vi "Stepper.vi"(0 "VISA resource name":refnum<visa-resource-name>="COM1", 1 "baud rate":u32=9600, 2 "data bits":u16=8 min=5 max=8 step=1, 3 "parity":u16(ring) items=["None", "Odd", "Even", "Mark", "Space"], 4 "stop bits":u16(ring)=10 items=["1.0"=10, "1.5"=15, "2.0"=20], 7 "flow control":u16(ring) items=["None"=0, "XON/XOFF"=1, "RTS/CTS"=2, "DTR/DSR"=4]) -> ()   [LabVIEW 2015]
doc: "The Basic Serial Read and Write example performs a Serial Port Read, a Serial Port Write, or a combination of these actions. The user selects the actions (read or write) on the front panel. If both are selected, the VI will write the data first, read data, and then close the VISA session that is opened to the port. This VI will wait until the specified number of bytes is received at the port. Only the number of bytes specified will be read.\n\nINSTRUCTIONS:\n1) Select the serial resource and configuration parameters (baud rate, data bits, parity, stop bits, flow control).\n2) Select the operations to be performed. \n3) Connect the serial port to your device. If no device is available, perform a loopback test by doing one of the following. Short pins 2 and 3 on a RS-232 cable or short pin 4 to pin 8 and pin 5 to pin 9 on a RS-485/422 cable. \n4) Run the VI to see the data read. (The \"read string\" will match the \"string to write\" if a loopback test was performed.)\n\nNote: The parameters set for the serial port must match the parameters of the connected instrument or device. In this example, the bytes to read parameter specifies the number of bytes that the serial port reads. If there were more bytes at the port than the number specified in bytes to read, those bytes would not be read. Also, if you specify to read more bytes than the number of bytes actually read, you might receive a timeout error message.\n\nOn the block diagram, the Configure Serial Port VI sets the configuration parameters. The front panel displays the controls used to configure the basic parameters, such as baud rate, data bits, and parity. Constants configure the other parameters the user probably does not need set. After the VISA Configure Serial Port VI opens the VISA session and configures the port, the VI passes the VISA resource name to other VIs that perform operations on that VISA resource. The VISA Write function sends a command to the serial device and the VISA Read function returns data based on the command. The VISA Close function then closes the reference to the serial device. It is important to close the reference; otherwise communication through with that port through protocols other than VISA might not be possible."
uses:
  <vilib>/Instr/_visa.llb/VISA Configure Serial Port (Instr).vi
panel:
  in  "?":string
  in  "Enable":bool
  in  "Clear 6":bool
  in  "Stop All":bool
  in  "Clear 5":bool
  in  "Direction 2":bool
  in  "Clear 4":bool
  in  "Direction 1":bool
  in  "Clear 3":bool
  in  "1/2  Step":bool
  in  "Clear 2":bool
  in  "Clear 1":bool
  in  "1/4 Step":bool
  in  "Reset The System":bool
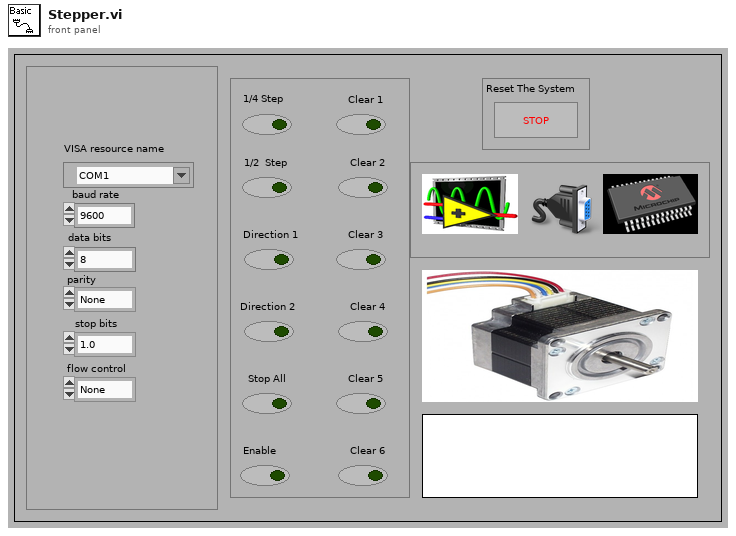
[diagram p1: front panel]
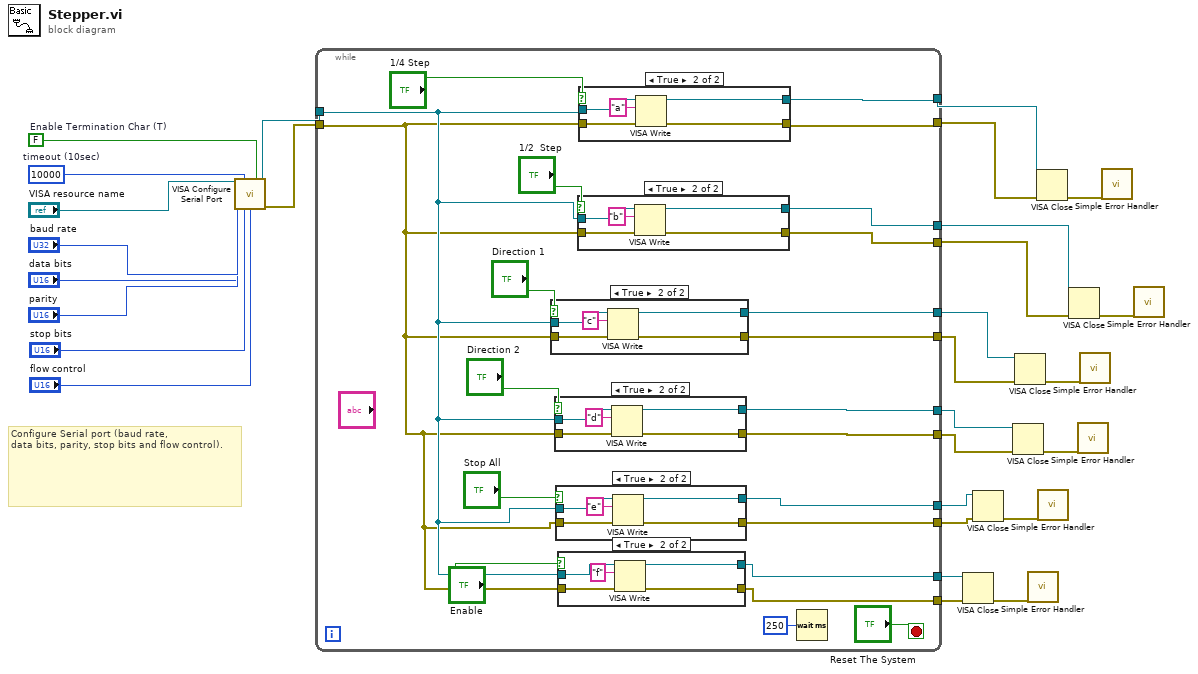
[diagram p0: block diagram]
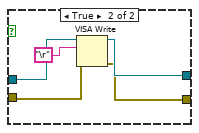
[diagram p3: hidden frame]
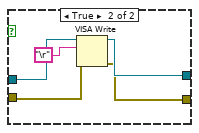
[diagram p5: hidden frame]
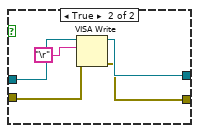
[diagram p7: hidden frame]
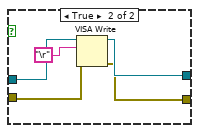
[diagram p9: hidden frame]
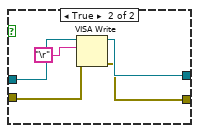
[diagram p11: hidden frame]
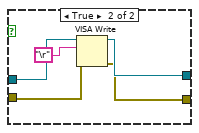
[diagram p13: hidden frame]
diagram:
  w21 = FALSE  # Enable Termination Char (T)
  w22 = u32 10000  # timeout (10sec)
  # "Configure Serial port (baud rate,\ndata bits, parity, stop bits and flow control)."
  n1 = call-poly "VISA Configure Serial Port"("VISA resource name"="VISA resource name", "timeout (10sec)"=w22, "Enable Termination\nChar (T)"=w21, "baud rate (9600)"="baud rate", "data bits (8)"="data bits", "parity (0:none)"="parity", "stop bits (10: 1 bit)"="stop bits", "flow control (0:none)"="flow control") -> ("VISA resource name out"=w25:refnum<visa-resource-name>, "error out"=w26:errorcluster)  [unwired: 6 in]
  n2 = while {
    tunnel: w26 -> [w33]
    tunnel: w25 -> [w34]
    tunnel: [w45] -> w17
    tunnel: [w47] -> w16
    tunnel: [w44] -> w14
    tunnel: [w43] -> w13
    tunnel: [w40] -> w10
    tunnel: [w39] -> w9
    tunnel: [w38] -> w8
    tunnel: [w37] -> w7
    tunnel: [w32] -> w4
    tunnel: [w31] -> w3
    tunnel: [w30] -> w2
    tunnel: [w29] -> w1
    stop <- "Reset The System" stop-if-true
    n3 = case shown="True" "Direction 1" {
      tunnel: [w102 w118] -> w40
      tunnel: w34 -> [w104 w117]
      tunnel: w33 -> [w105 w115]
      tunnel: [w103 w116] -> w39
      frame False {
        n4 = case shown="False" "Clear 3" {
          tunnel: w105 -> [w107 w113]
          tunnel: w104 -> [w108 w112]
          tunnel: [w108 w110] -> w103
          tunnel: [w107 w109] -> w102
          frame False {
          }
          frame True {
            n5 = VISA Write(VISA resource name=w112, write buffer="\r", error in (no error)=w113) -> (VISA resource name out=w110:refnum<visa-resource-name>, error out=w109:errorcluster)  [unwired: 1 out]
          }
        }
      }
      frame True {
        n6 = VISA Write(VISA resource name=w117, write buffer="c", error in (no error)=w115) -> (VISA resource name out=w116:refnum<visa-resource-name>, error out=w118:errorcluster)  [unwired: 1 out]
      }
    }
    n7 = case shown="True" "Direction 2" {
      tunnel: [w85 w101] -> w37
      tunnel: w34 -> [w87 w100]
      tunnel: w33 -> [w88 w98]
      tunnel: [w86 w99] -> w38
      frame False {
        n8 = case shown="False" "Clear 4" {
          tunnel: w88 -> [w90 w96]
          tunnel: w87 -> [w91 w95]
          tunnel: [w91 w93] -> w86
          tunnel: [w90 w92] -> w85
          frame False {
          }
          frame True {
            n9 = VISA Write(VISA resource name=w95, write buffer="\r", error in (no error)=w96) -> (VISA resource name out=w93:refnum<visa-resource-name>, error out=w92:errorcluster)  [unwired: 1 out]
          }
        }
      }
      frame True {
        n10 = VISA Write(VISA resource name=w100, write buffer="d", error in (no error)=w98) -> (VISA resource name out=w99:refnum<visa-resource-name>, error out=w101:errorcluster)  [unwired: 1 out]
      }
    }
    n11 = case shown="True" "Stop All" {
      tunnel: [w51 w67] -> w31
      tunnel: w34 -> [w53 w66]
      tunnel: w33 -> [w54 w64]
      tunnel: [w52 w65] -> w32
      frame False {
        n12 = case shown="False" "Clear 5" {
          tunnel: w54 -> [w56 w62]
          tunnel: w53 -> [w57 w61]
          tunnel: [w57 w59] -> w52
          tunnel: [w56 w58] -> w51
          frame False {
          }
          frame True {
            n13 = VISA Write(VISA resource name=w61, write buffer="\r", error in (no error)=w62) -> (VISA resource name out=w59:refnum<visa-resource-name>, error out=w58:errorcluster)  [unwired: 1 out]
          }
        }
      }
      frame True {
        n14 = VISA Write(VISA resource name=w66, write buffer="e", error in (no error)=w64) -> (VISA resource name out=w65:refnum<visa-resource-name>, error out=w67:errorcluster)  [unwired: 1 out]
      }
    }
    n15 = case shown="True" "Enable" {
      tunnel: [w68 w84] -> w29
      tunnel: w34 -> [w70 w83]
      tunnel: w33 -> [w71 w81]
      tunnel: [w69 w82] -> w30
      frame False {
        n16 = case shown="False" "Clear 6" {
          tunnel: w71 -> [w73 w79]
          tunnel: w70 -> [w74 w78]
          tunnel: [w74 w76] -> w69
          tunnel: [w73 w75] -> w68
          frame False {
          }
          frame True {
            n17 = VISA Write(VISA resource name=w78, write buffer="\r", error in (no error)=w79) -> (VISA resource name out=w76:refnum<visa-resource-name>, error out=w75:errorcluster)  [unwired: 1 out]
          }
        }
      }
      frame True {
        n18 = VISA Write(VISA resource name=w83, write buffer="f", error in (no error)=w81) -> (VISA resource name out=w82:refnum<visa-resource-name>, error out=w84:errorcluster)  [unwired: 1 out]
      }
    }
    n19 = case shown="True" "1/2  Step" {
      tunnel: [w119 w135] -> w43
      tunnel: w34 -> [w121 w134]
      tunnel: w33 -> [w122 w132]
      tunnel: [w120 w133] -> w44
      frame False {
        n20 = case shown="False" "Clear 2" {
          tunnel: w122 -> [w124 w130]
          tunnel: w121 -> [w125 w129]
          tunnel: [w125 w127] -> w120
          tunnel: [w124 w126] -> w119
          frame False {
          }
          frame True {
            n21 = VISA Write(VISA resource name=w129, write buffer="\r", error in (no error)=w130) -> (VISA resource name out=w127:refnum<visa-resource-name>, error out=w126:errorcluster)  [unwired: 1 out]
          }
        }
      }
      frame True {
        n22 = VISA Write(VISA resource name=w134, write buffer="b", error in (no error)=w132) -> (VISA resource name out=w133:refnum<visa-resource-name>, error out=w135:errorcluster)  [unwired: 1 out]
      }
    }
    n23 = case shown="True" "1/4 Step" {
      tunnel: [w136 w152] -> w47
      tunnel: w34 -> [w138 w151]
      tunnel: w33 -> [w139 w149]
      tunnel: [w137 w150] -> w45
      frame False {
        n24 = case shown="False" "Clear 1" {
          tunnel: w139 -> [w141 w147]
          tunnel: w138 -> [w142 w146]
          tunnel: [w142 w144] -> w137
          tunnel: [w141 w143] -> w136
          frame False {
          }
          frame True {
            n25 = VISA Write(VISA resource name=w146, write buffer="\r", error in (no error)=w147) -> (VISA resource name out=w144:refnum<visa-resource-name>, error out=w143:errorcluster)  [unwired: 1 out]
          }
        }
      }
      frame True {
        n26 = VISA Write(VISA resource name=w151, write buffer="a", error in (no error)=w149) -> (VISA resource name out=w150:refnum<visa-resource-name>, error out=w152:errorcluster)  [unwired: 1 out]
      }
    }
    n27 = Wait (ms)(milliseconds to wait=u32 250) -> ()  [unwired: 1 out]
  }
  n28 = VISA Close(VISA resource name=w2, error in (no error)=w1) -> (error out=w5:errorcluster)
  n29 = VISA Close(VISA resource name=w4, error in (no error)=w3) -> (error out=w6:errorcluster)
  n30 = VISA Close(VISA resource name=w8, error in (no error)=w7) -> (error out=w11:errorcluster)
  n31 = VISA Close(VISA resource name=w9, error in (no error)=w10) -> (error out=w12:errorcluster)
  n32 = call <vilib>:"Simple Error Handler.vi"("error in (no error)"=w5) -> ()  [unwired: 4 in, 5 out]
  n33 = VISA Close(VISA resource name=w17, error in (no error)=w16) -> (error out=w24:errorcluster)
  n34 = call <vilib>:"Simple Error Handler.vi"("error in (no error)"=w6) -> ()  [unwired: 4 in, 5 out]
  n35 = VISA Close(VISA resource name=w14, error in (no error)=w13) -> (error out=w15:errorcluster)
  n36 = call <vilib>:"Simple Error Handler.vi"("error in (no error)"=w11) -> ()  [unwired: 4 in, 5 out]
  n37 = call <vilib>:"Simple Error Handler.vi"("error in (no error)"=w12) -> ()  [unwired: 4 in, 5 out]
  n38 = call <vilib>:"Simple Error Handler.vi"("error in (no error)"=w24) -> ()  [unwired: 4 in, 5 out]
  n39 = call <vilib>:"Simple Error Handler.vi"("error in (no error)"=w15) -> ()  [unwired: 4 in, 5 out]
